vi "1radar.vi"(7 "date/time string":string, 8 "Q":dbl[](array[numeric]), 9 "I":dbl[](array[numeric]), 10 "radar number":i32, 11 "input cluster":T1) -> (0 "error out":errorcluster, 1 "Q out":dbl[](array[numeric]), 2 "I out":dbl[](array[numeric]), 3 "VISA resource out":refnum<visa-resource-name>, 4 "Spectrum":waveform(dbl)(graph), 5 "I/Q channels":dynamicdata(graph))   [LabVIEW 2015]
uses:
  <vilib>/Analysis/2dsp.llb/Complex FFT.vi
  <vilib>/measure/madcrms.llb/Basic Averaged DC-RMS for 1 Chan.vi
  <vilib>/measure/NI_MAPro.lvlib
  <vilib>/Analysis/NI_AALPro.lvlib
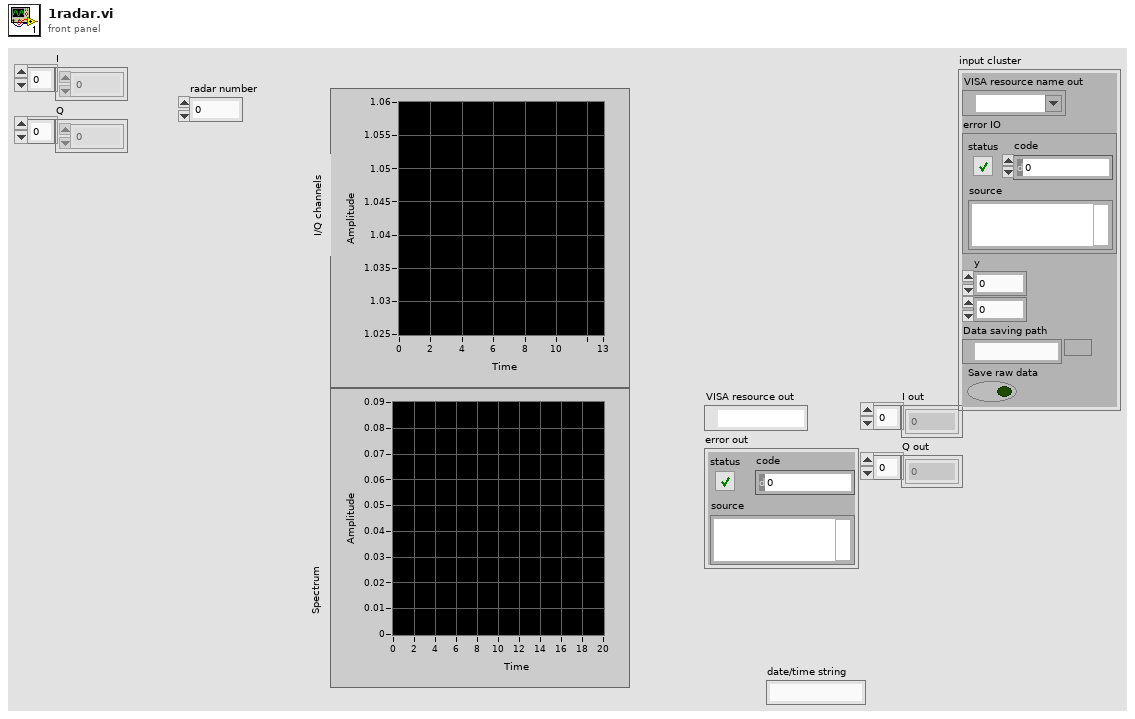
[diagram p1: front panel]
types:
  T1 = cluster{"VISA resource name out":refnum<visa-resource-name>, "error IO":errorcluster, "y":u8, i32, "Data saving path":path, "Save raw data":bool}
  T2 = enum16{"open", "replace", "create", "open or create", "replace or create", "replace or create with confirmation"}
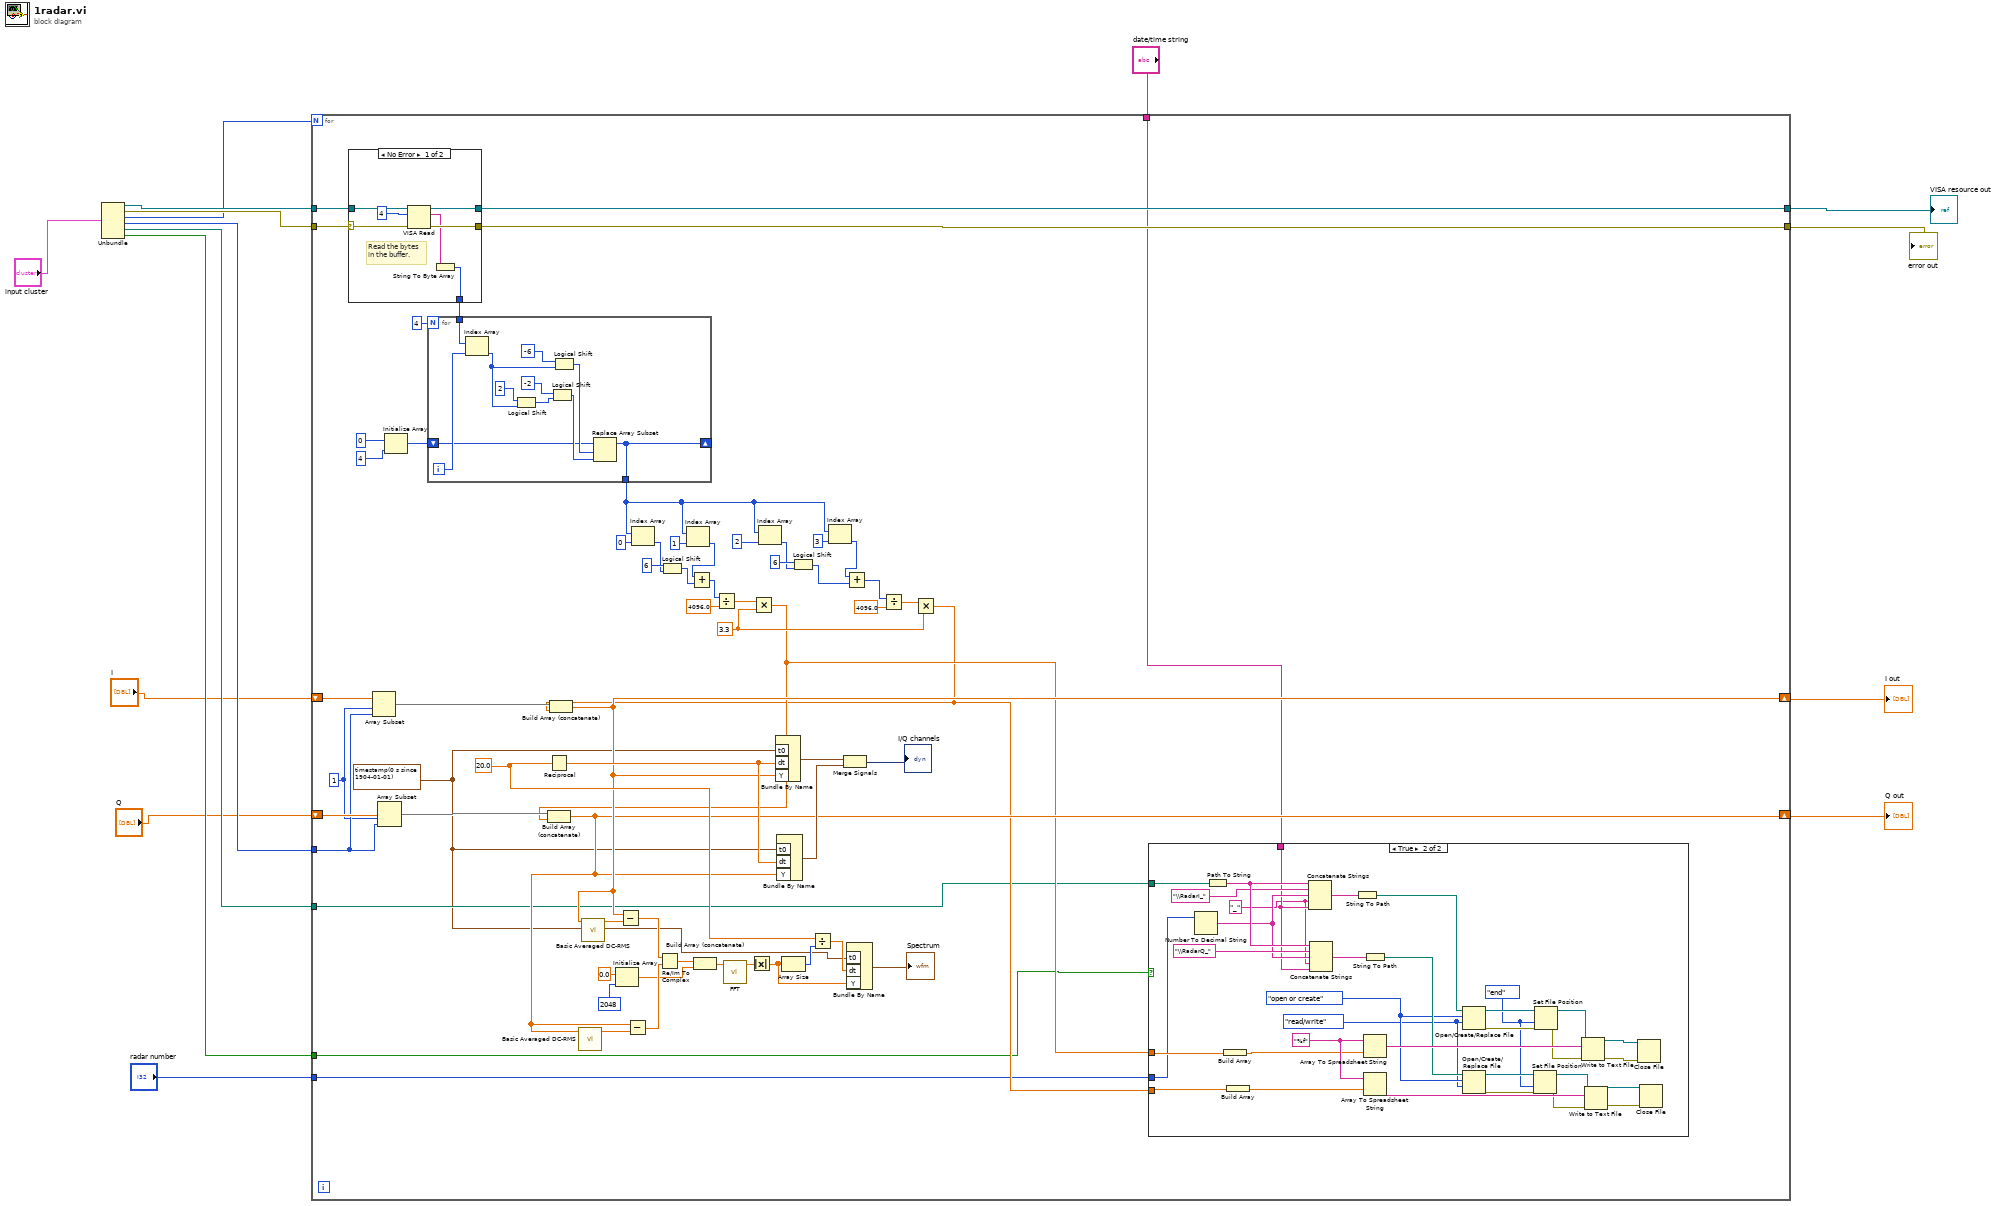
[diagram p0: block diagram]
diagram:
  n1 = Unbundle("input cluster") -> ("VISA resource name out"=w10:refnum<visa-resource-name>, "error IO"=w9:errorcluster, "y"=w6:u8, w5:i32, "Data saving path"=w4:path, "Save raw data"=w3:bool)
  n2 = for {
    N: w6 -> [_]
    tunnel: w9 -> [w50]
    tunnel: w10 -> [w49]
    tunnel: [w25] -> w14
    tunnel: [w24] -> w13
    tunnel: w5 -> [w62]
    shift-right: [w30] -> w11
    shift-left: "Q" -> [w77]
    shift-right: [w31] -> w12
    shift-left: "I" -> [w63]
    tunnel: "date/time string" -> [w22]
    tunnel: "radar number" -> [w19]
    tunnel: w4 -> [w18]
    tunnel: w3 -> [w17]
    w16 = timestamp(0 s since 1904-01-01) ("t0")
    w32 = 1 ("index")
    (unwired) 0
    w55 = 3.3 ("y")
    w39 = 20.0 ("dt")
    n3 = case "Read bytes from port." shown="No Error" w50 {
      selector: w50 -> [w127 w132]
      tunnel: [w129 w132] -> w24
      tunnel: [w130 w133] -> w25
      tunnel: w49 -> [w128 w133]
      tunnel: [w125 u8[] [] ("unsigned byte array")] -> w26
      frame No Error {
        # "Read the bytes\nin the buffer."
        n4 = VISA Read(VISA resource name=w128, byte count=u32 4, error in (no error)=w127) -> (VISA resource name out=w130:refnum<visa-resource-name>, read buffer=w126:string, error out=w129:errorcluster)  [unwired: 1 out]
        n5 = String To Byte Array(string=w126) -> (unsigned byte array=w125:u8[])
      }
      frame Error {
        # "Error occurred \nreading Bytes at \nSerial Port"
      }
    }
    n6 = Array Subset(array=w63, index=w32, length=w62) -> (w64:dbl[])
    n7 = Array Subset(array=w77, index=w32, length=w62) -> (w78:dbl[])
    n8 = Initialize Array(i16 0 ("element"), 4 ("dimension size")) -> (w27:i16[])
    n9 = for {
      N: 4 -> [_]
      tunnel: w26 -> [w118]
      tunnel: [w113] -> w33
      shift-right: [w113] -> _
      shift-left: w27 -> [w114]
      i -> [w117]
      n10 = Index Array(array=w118, index=w117) -> (element=w121:u8)
      n11 = Logical Shift(y=i8 2, x=w121) -> (x << y=w120:u8)
      n12 = Logical Shift(y=i8 -2, x=w120) -> (x << y=w115:u8)
      n13 = Logical Shift(y=i8 -6, x=w121) -> (x << y=w116:u8)
      n14 = Replace Array Subset(array=w114, new element=w115, index=w116) -> (w113:i16[])
    }
    n15 = Reciprocal(x=w39) -> (1/x=w53:dbl)
    n16 = Initialize Array(0.0 ("element"), 2048 ("dimension size")) -> (w43:dbl[])
    n17 = Index Array(array=w33, index=0) -> (element=w71:i16)
    n18 = Logical Shift(y=i16 6, x=w71) -> (x << y=w67:i16)
    n19 = Index Array(array=w33, index=1) -> (element=w68:i16)
    n20 = Add(x=w68, y=w67) -> (x+y=w23:i16)
    n21 = Divide(x=w23, y=4096.0) -> (x/y=w60:dbl)
    n22 = Multiply(x=w60, y=w55) -> (x*y=w21:dbl)
    n23 = Build Array (concatenate)(w78, w21) -> (w30:dbl[])
    n24 = call-poly <vilib>:"Basic Averaged DC-RMS.vi"("signal in"=w30) -> ("DC value"=w56:dbl)  [unwired: 4 in, 6 out]
    n25 = Subtract(x=w30, y=w56) -> (x-y=w47:dbl[])
    n26 = Index Array(array=w33, index=2) -> (element=w69:i16)
    n27 = Bundle By Name ("Build Waveform")("t0"=w16, "dt"=w53, "Y"=w30) -> (w51:waveform(dbl))  [unwired: 1 out]
    n28 = Logical Shift(y=i16 6, x=w69) -> (x << y=w65:i16)
    n29 = Index Array(array=w33, index=3) -> (element=w66:i16)
    n30 = Add(x=w66, y=w65) -> (x+y=w35:i16)
    n31 = Divide(x=w35, y=4096.0) -> (x/y=w58:dbl)
    n32 = Multiply(x=w58, y=w55) -> (x*y=w20:dbl)
    n33 = Build Array (concatenate)(w64, w20) -> (w31:dbl[])
    n34 = call-poly <vilib>:"Basic Averaged DC-RMS.vi"("signal in"=w31) -> ("DC value"=w57:dbl)  [unwired: 4 in, 6 out]
    n35 = Subtract(x=w31, y=w57) -> (x-y=w48:dbl[])
    n36 = Re/Im To Complex(1:w47, 2:w48) -> (0:w42:cdb[])
    n37 = Build Array (concatenate)(w42, w43) -> (w44:cdb[])
    n38 = call-poly <vilib>:"FFT.vi"("X"=w44) -> ("FFT {X}"=w40:cdb[])  [unwired: 2 in, 8 out]
    n39 = Absolute Value(x=w40) -> (abs(x)=w38:dbl[])
    n40 = Bundle By Name ("Build Waveform")("t0"=w16, "dt"=w53, "Y"=w31) -> (w52:waveform(dbl))  [unwired: 1 out]
    n41 = Array Size(array=w38) -> (size(s)=w41:i32)
    n42 = Divide(x=w39, y=w41) -> (x/y=w37:dbl)
    n43 = Merge Signals(w52, w51) -> (→"I/Q channels":dynamicdata)
    n44 = Bundle By Name("t0"=w16, "dt"=w37, "Y"=w38) -> (→"Spectrum":waveform(dbl))  [unwired: 1 out]
    n45 = case shown="True" w17 {
      tunnel: w21 -> [_ w103]
      tunnel: w20 -> [_ w84]
      tunnel: w22 -> [_ w81]
      tunnel: w18 -> [_ w104]
      tunnel: w19 -> [_ w80]
      frame False {
      }
      frame True {
        w79 = "_" ("string")
        w85 = enum16{"read/write", "read-only", "write-only"}."read/write" ("access (0:read/write)")
        w86 = T2."open or create" ("operation (0:open)")
        w94 = enum16{"start", "end", "current"}."end" ("from (0:start)")
        w108 = "%f" ("format string")
        n46 = Number To Decimal String(number=w80) -> (decimal integer string=w82:string)  [unwired: 1 in]
        n47 = Path To String(path=w104) -> (string=w110:string)
        n48 = Build Array(w103) -> (w83:dbl[])
        n49 = Build Array(w84) -> (w102:dbl[])
        n50 = Concatenate Strings(w110, "\\RadarI_" ("string"), w82, w79, w81) -> (w112:string)
        n51 = Concatenate Strings(w110, "\\RadarQ_" ("string"), w82, w79, w81) -> (w109:string)
        n52 = String To Path(string=w112) -> (path=w101:path)
        n53 = Array To Spreadsheet String(array=w83, 3:w108) -> (spreadsheet string=w111:string)  [unwired: 1 in]
        n54 = Array To Spreadsheet String(array=w102, 3:w108) -> (spreadsheet string=w107:string)  [unwired: 1 in]
        n55 = String To Path(string=w109) -> (path=w100:path)
        n56 = Open/Create/Replace File(file path (use dialog)=w101, operation (0:open)=w86, access (0:read/write)=w85) -> (refnum out=w99:refnum<file>, error out=w98:errorcluster)  [unwired: 3 in, 1 out]
        n57 = Open/Create/Replace File(file path (use dialog)=w100, operation (0:open)=w86, access (0:read/write)=w85) -> (refnum out=w95:refnum<file>, error out=w93:errorcluster)  [unwired: 3 in, 1 out]
        n58 = Set File Position(refnum=w95, from (0:start)=w94, error in=w93) -> (refnum out=w91:refnum<file>, error out=w92:errorcluster)  [unwired: 1 in]
        n59 = Set File Position(refnum=w99, from (0:start)=w94, error in=w98) -> (refnum out=w97:refnum<file>, error out=w96:errorcluster)  [unwired: 1 in]
        n60 = Write to Text File(file (use dialog)=w97, text=w111, error in=w96) -> (refnum out=w90:refnum<file>, error out=w89:errorcluster)  [unwired: 1 in, 1 out]
        n61 = Write to Text File(file (use dialog)=w91, text=w107, error in=w92) -> (refnum out=w88:refnum<file>, error out=w87:errorcluster)  [unwired: 1 in, 1 out]
        n62 = Close File(refnum=w90, error in=w89) -> ()  [unwired: 2 out]
        n63 = Close File(refnum=w88, error in=w87) -> ()  [unwired: 2 out]
      }
    }
  }
  "VISA resource out" <- w14
  "error out" <- w13
  "I out" <- w12
  "Q out" <- w11
